vi "Launcher.vi"() -> ()   [LabVIEW 2018]
panel:
  in  "IconEditor 5":bool caption="空白按钮"
  in  "IconEditor 4":bool caption="空白按钮"
  in  "IconEditor 3":bool caption="空白按钮"
  in  "preset":bool caption="空白按钮"
  in  "IconEditor":bool caption="空白按钮"
  in  "VIAttribution":bool caption="空白按钮"
  in  "TerminalSet":bool caption="空白按钮"
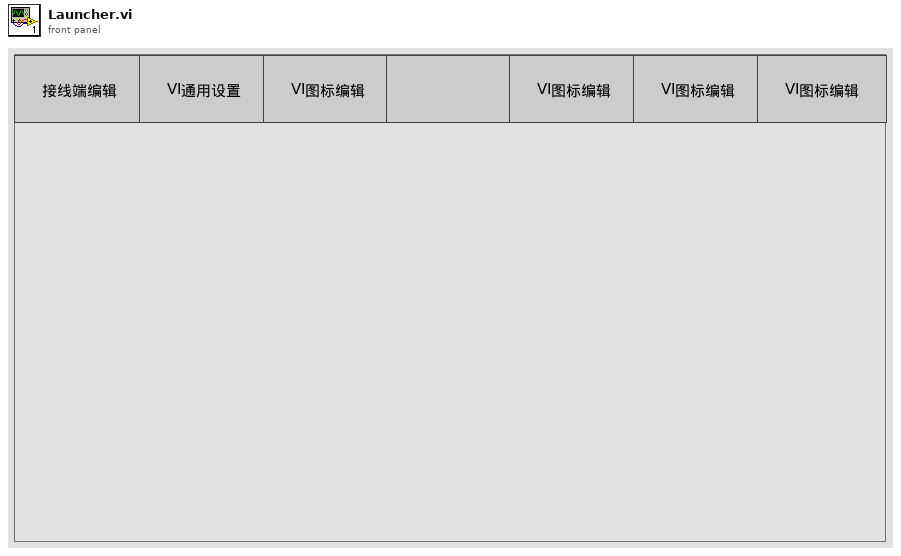
[diagram p1: front panel]
types:
  T1 = enum32{"Invalid", "Standard", "Closed", "Hidden", "Minimized", "Maximized"}
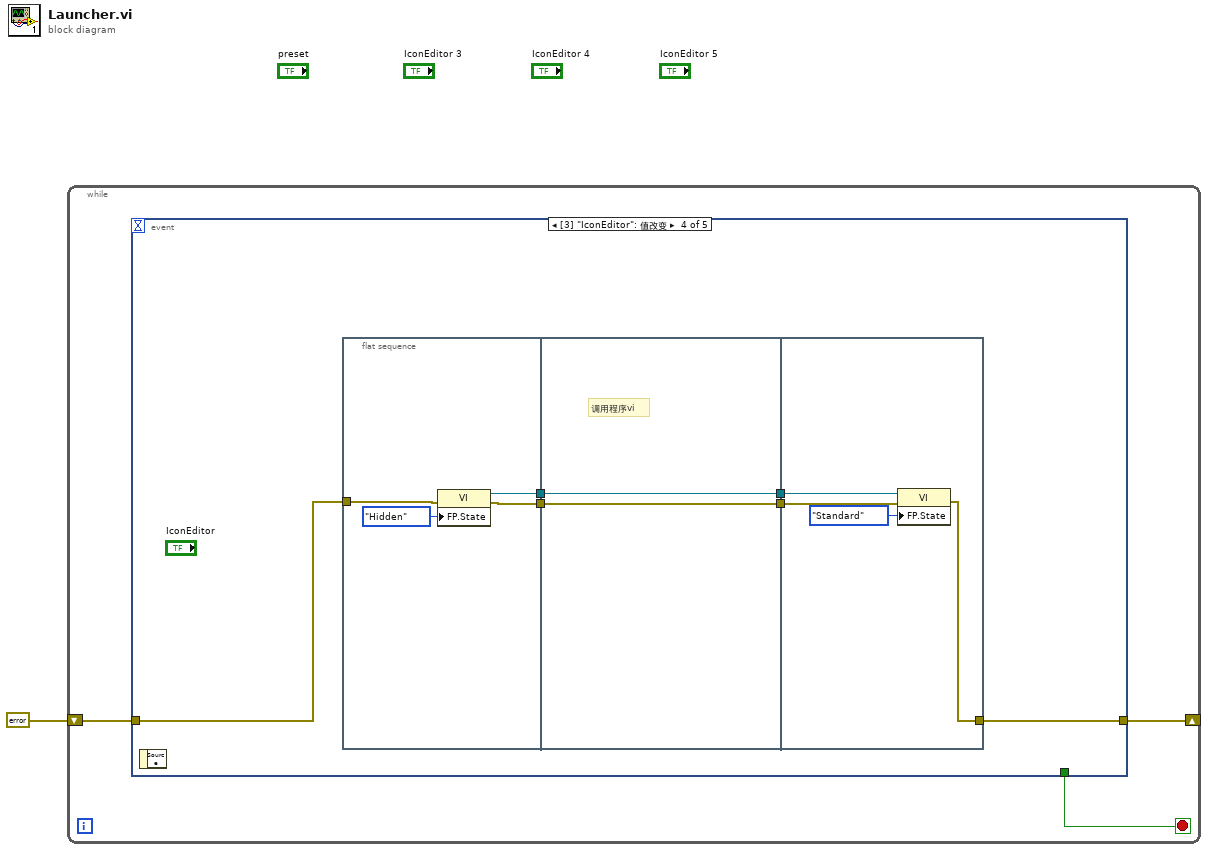
[diagram p0: block diagram]
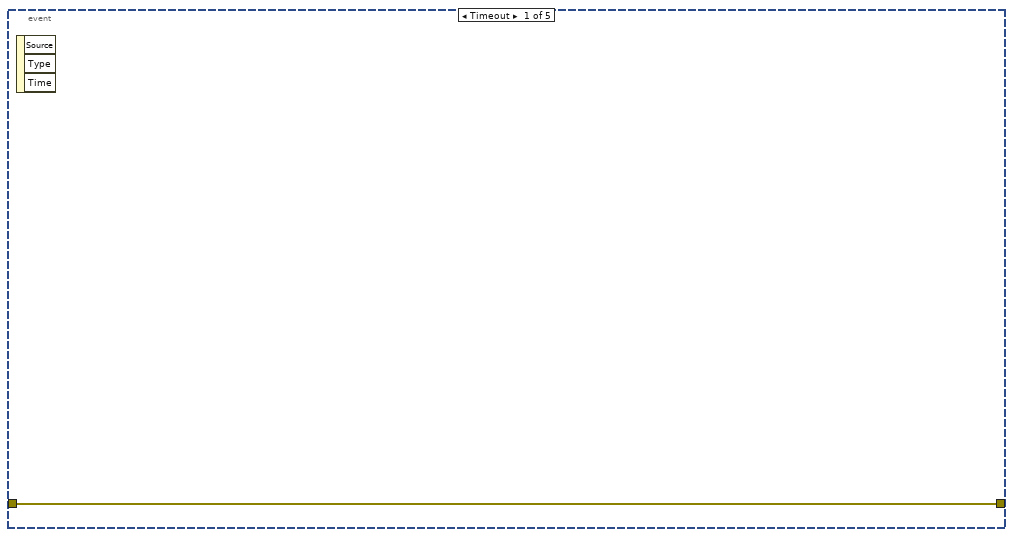
[diagram p2: hidden frame]
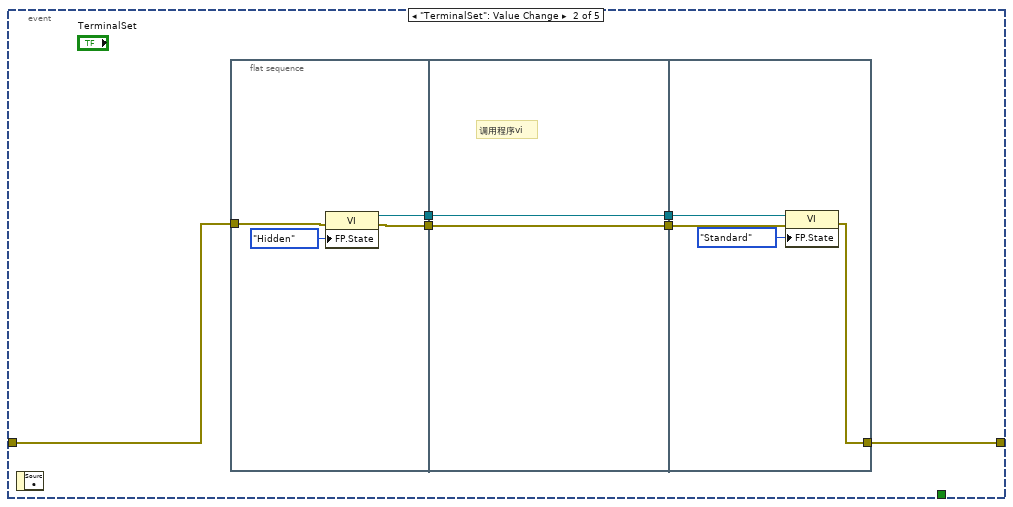
[diagram p3: hidden frame]
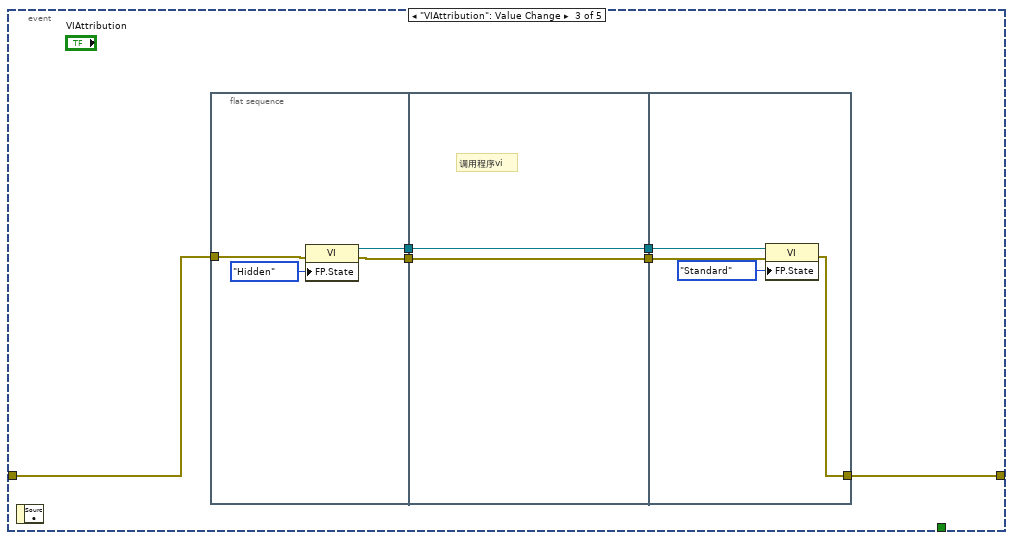
[diagram p4: hidden frame]
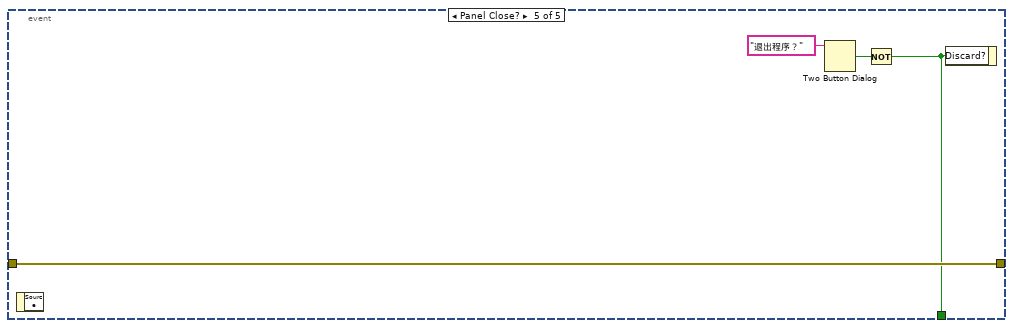
[diagram p5: hidden frame]
diagram:
  n1 = while {
    shift-right: [w3] -> _
    shift-left: errorcluster {"status"=FALSE, "code"=0, "source"=""} ("错误常量") -> [w4]
    stop <- w2 stop-if-true
    n2 = event shown="[3] \"IconEditor\": 值改变" {
      selector: _ -> [_ _ _ _ _]
      dyn-events: _ -> [_ _ _ _ _]
      timeout: _ -> [_ _ _ _ _]
      tunnel: w4 -> [w5 w11 w23 w38 w55]
      tunnel: [w5 w6 w22 w39 w55] -> w3
      tunnel: [_ _ _ _ w54] -> w2
      event Timeout {
        n3 = event-data() -> ()  [unwired: 1 in, 3 out]
      }
      event "TerminalSet": Value Change {
        n4 = event-data() -> ()  [unwired: 1 in, 1 out]
        n5 = flat-sequence {
          tunnel: w11 -> [w14]
          tunnel: [w13] -> w10
          tunnel: [w12] -> w8
          tunnel: w10 -> [w17]
          tunnel: [w17] -> w9
          tunnel: w8 -> [w16]
          tunnel: [w16] -> w7
          tunnel: w9 -> [w21]
          tunnel: w7 -> [w20]
          tunnel: [w18] -> w6
          frame #0 {
            n6 = property class="VI"(error in=w14, "FP.State"=T1."Hidden" ("前面板窗口:状态")) -> (reference out=w13:refnum<vi>, error out=w12:errorcluster)  [unwired: 1 in]
          }
          frame #1 {
            # "调用程序vi"
          }
          frame #2 {
            n7 = property class="VI"(reference=w21, error in=w20, "FP.State"=T1."Standard" ("前面板窗口:状态")) -> (error out=w18:errorcluster)  [unwired: 1 out]
          }
        }
      }
      event "VIAttribution": Value Change {
        n8 = event-data() -> ()  [unwired: 1 in, 1 out]
        n9 = flat-sequence {
          tunnel: w23 -> [w30]
          tunnel: [w29] -> w27
          tunnel: [w28] -> w26
          tunnel: w27 -> [w33]
          tunnel: [w33] -> w25
          tunnel: w26 -> [w32]
          tunnel: [w32] -> w24
          tunnel: w25 -> [w37]
          tunnel: w24 -> [w36]
          tunnel: [w34] -> w22
          frame #0 {
            n10 = property class="VI"(error in=w30, "FP.State"=T1."Hidden" ("前面板窗口:状态")) -> (reference out=w29:refnum<vi>, error out=w28:errorcluster)  [unwired: 1 in]
          }
          frame #1 {
            # "调用程序vi"
          }
          frame #2 {
            n11 = property class="VI"(reference=w37, error in=w36, "FP.State"=T1."Standard" ("前面板窗口:状态")) -> (error out=w34:errorcluster)  [unwired: 1 out]
          }
        }
      }
      event "IconEditor": Value Change {
        n12 = event-data() -> ()  [unwired: 1 in, 1 out]
        n13 = flat-sequence {
          tunnel: w38 -> [w46]
          tunnel: [w45] -> w43
          tunnel: [w44] -> w42
          tunnel: w43 -> [w49]
          tunnel: [w49] -> w41
          tunnel: w42 -> [w48]
          tunnel: [w48] -> w40
          tunnel: w41 -> [w53]
          tunnel: w40 -> [w52]
          tunnel: [w50] -> w39
          frame #0 {
            n14 = property class="VI"(error in=w46, "FP.State"=T1."Hidden" ("前面板窗口:状态")) -> (reference out=w45:refnum<vi>, error out=w44:errorcluster)  [unwired: 1 in]
          }
          frame #1 {
            # "调用程序vi"
          }
          frame #2 {
            n15 = property class="VI"(reference=w53, error in=w52, "FP.State"=T1."Standard" ("前面板窗口:状态")) -> (error out=w50:errorcluster)  [unwired: 1 out]
          }
        }
      }
      event Panel Close? {
        n16 = event-data() -> ()  [unwired: 1 in, 1 out]
        n17 = Two Button Dialog(message="退出程序？" ("消息")) -> (T button?=w56:bool)  [unwired: 2 in]
        n18 = Not(x=w56) -> (.not. x?=w54:bool)
        n19 = event-data("Discard?"=w54) -> ()  [unwired: 1 in, 1 out]
      }
    }
  }
